vi "analyze_raw_data.vi"() -> ()   [LabVIEW 2017]
uses:
  <vilib>/Utility/file.llb/Read Delimited Spreadsheet (I64).vi
panel:
  out "Array":i64[][](array[numeric])
  in  "ch list":u16[](array[numeric])=[0, 1, 6, 7]
  in  "file path (dialog if empty)":path=path "E:/tdc/2017/test_20240319_042405_codeDensity.csv"
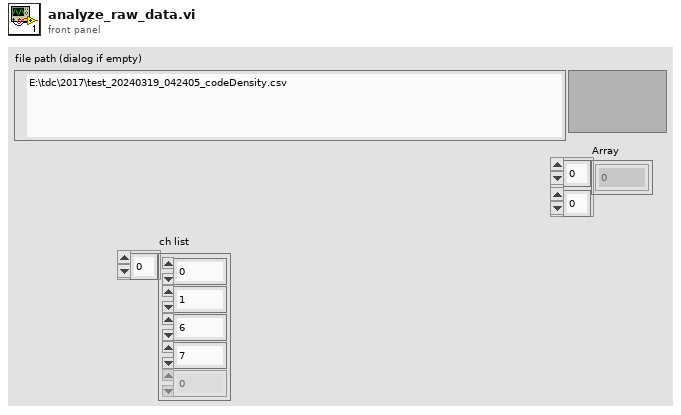
[diagram p1: front panel]
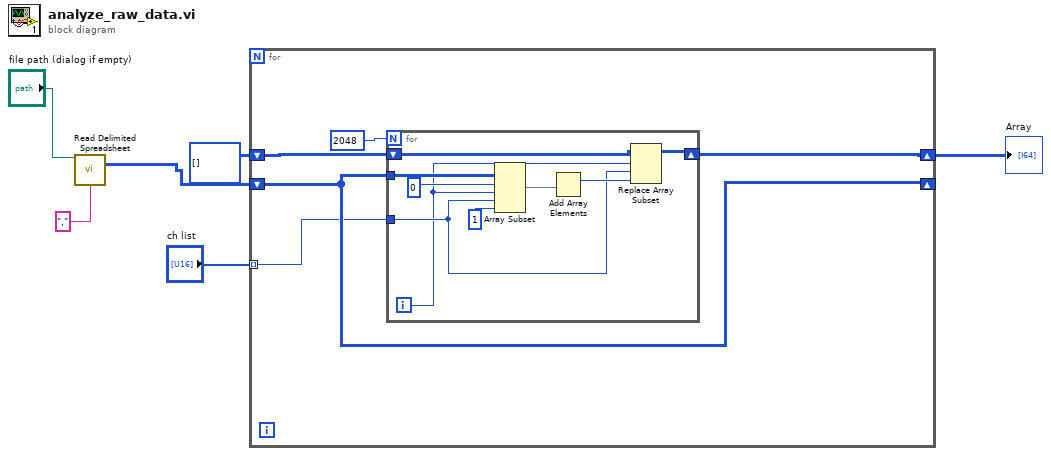
[diagram p0: block diagram]
diagram:
  n1 = call-poly <vilib>:"Read Delimited Spreadsheet.vi"("file path (dialog if empty)"="file path (dialog if empty)", "delimiter (\\t)"="," ("delimiter (\\t)")) -> ("all rows"=w6:i64[][])  [unwired: 8 in, 5 out]
  n2 = for {
    shift-right: [w9] -> w1
    shift-left: i64[][] [] -> [w10]
    shift-right: [w8] -> _
    shift-left: w6 -> [w8]
    tunnel: "ch list" -> [w7] mode=indexing
    n3 = for {
      N: 2048 -> [_]
      tunnel: w8 -> [w20]
      tunnel: w7 -> [w13]
      shift-right: [w15] -> w9
      shift-left: w10 -> [w16]
      i -> [w12]
      n4 = Array Subset(array=w20, index (row)=0 ("索引"), length (row)=w12, index (col)=w13, length (col)=1 ("长度")) -> (w17:i64[][])
      n5 = Add Array Elements(numeric array=w17) -> (sum=w14:i64)
      n6 = Replace Array Subset(array=w16, new element=w14, index (row)=w12, index (col)=w13) -> (w15:i64[][])
    }
  }
  "Array" <- w1
